vi "Compute Counter Params.vi"(8 "error in (no error)":errorcluster, 10 "Trial duration (s)":dbl) -> (0 "error out":errorcluster)   [LabVIEW 2015]
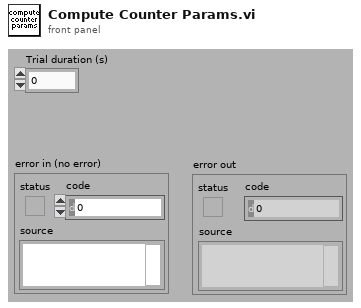
[diagram p1: front panel]
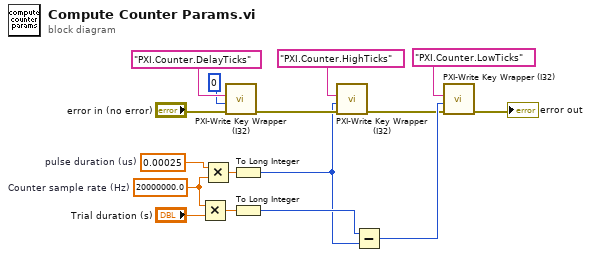
[diagram p0: block diagram]
diagram:
  w7 = 20000000.0  # Counter sample rate (Hz)
  w6 = 0.00025  # pulse duration (us)
  n1 = Multiply(x=w7, y="Trial duration (s)") -> (x*y=w10:dbl)
  n2 = Multiply(x=w6, y=w7) -> (x*y=w5:dbl)
  n3 = call "PXI-Write Key Wrapper (I32).vi"("error in (no error)"="error in (no error)", "value"=0, "key"="PXI.Counter.DelayTicks") -> ("error out"=w9:errorcluster)  [unwired: 8 in]
  n4 = To Long Integer(number=w5) -> (32bit integer=w3:i32)
  n5 = To Long Integer(number=w10) -> (32bit integer=w4:i32)
  n6 = call "PXI-Write Key Wrapper (I32).vi"("error in (no error)"=w9, "value"=w3, "key"="PXI.Counter.HighTicks") -> ("error out"=w2:errorcluster)  [unwired: 8 in]
  n7 = Subtract(x=w4, y=w3) -> (x-y=w12:i32)
  n8 = call "PXI-Write Key Wrapper (I32).vi"("error in (no error)"=w2, "value"=w12, "key"="PXI.Counter.LowTicks") -> ("error out"=→"error out":errorcluster)  [unwired: 8 in]
